vi "pulse_ring_averager.vi"() -> ()   [LabVIEW 2014]
uses:
  <vilib>/express/express analysis/Spectral/Block/exnSpectralBlock spectral measurements RMS poly.vi
  <vilib>/express/express analysis/Spectral/Block/exnSpectralBlock spectral measurements RMS WFM.vi
  <vilib>/Utility/file.llb/Write To Spreadsheet File (DBL).vi
  <vilib>/express/express analysis/Spectral/XNode/ExpressSpectralMeasurementsBlockNode.xnode
panel:
  in  "Create Spreadsheet Data?":bool
  in  "?":bool
  out "Waveform Graph":cluster{"f0":dbl, "df":dbl, "magnitude":dbl[]}(graph)={"f0"=0.0, "df"=5.0, "magnitude"=[8.352033063743602e-05, 0.0001521936782107742, 0.0001241645669166561, 0.0005913924283974822, 0.0017924539602640116, 0.002361467917160108, 0.0013264978014836787, 0.0008901875481831404, 0.00073723890923067, 0.0003785453068588639, 0.0001836739230249787, 3.197394988898929e-05, 0.00023707241273739638, 0.00018007989851456744, 4.770297439969988e-05, 0.0001260879375301181, 0.00011358993968053149, 9.416072191429606e-05, 2.3266024527903313e-05, 0.00014747301423229434, 0.00021873863503173966, 0.00016382863521811113, 0.00030989231903681013, 0.0006848998054862691, 0.0006929060488089187, 0.00011498969012903245, 0.0010445143273397997, 0.0021663414429004663, 0.0025925396298316, 0.0015150935560222308, 0.005327334532678184, 0.0233859554577817, 0.02859469559502763, 0.009897156395780392, 0.001793115328993954, 0.0005236696631654215, 0.0006446389975765783, 0.0018452938517409666, 0.0016391137319586276, 0.0005787100388248387, 0.0001698622098812452, 0.00016031383859121896, 9.318098751849772e-05, 4.9411270959326514e-05, 0.00018102626398632646, 0.0001772618334287019, 8.862654858080105e-05, 0.00010413603644766573, 4.065137938351173e-05, 6.325569194929935e-05, 3.7785144930814025e-05, 8.44451565632641e-05, 0.00011643844181054693, 0.00012102920589116524, 6.558259148383841e-05, 2.6563415271802513e-05, 9.419033683439217e-05, 0.00024452333927457243, 0.00021172954941749473, 0.00010011909206931354, 0.00040767861329374014, 0.00089963628760365, 0.0013620238335515452, 0.0033111439875997645, 0.003843956937129491, 0.0021381752402404365, 0.0006642447893147237, 0.0003523770956178529, 0.0009192108548157987, 0.00240667098631922, 0.003199856811538736, 0.0020968774819987443, 0.000781225449659328, 0.0012720686213830836, 0.0011307985420501722, 0.00041317105628617623, 5.672232242689178e-05, 0.00019255456754959516, 0.00016272162386009182, 3.994272788022854e-05, 2.911455610905325e-05, 4.3973070727008133e-05, 3.0127385533287327e-05, 5.478402759196668e-05, 7.214350960014323e-05, 0.00010803424524223192, 6.0967411444140105e-05, 5.142072772087622e-05, 4.857738287964089e-05, 0.000184071319208993, 0.00039623072384841645, 0.00037089595185725214, 0.000464718422038645, 0.0013054691711676788, 0.0015883351276961978, 0.0009090460049399212, 0.0010413359930296908, 0.0012816866380819423, 0.0010403077729971293, 0.0005914864424886577]}
  out "Dynamic Data Type":waveform(dbl)(graph)={"t0"=timestamp(0 s since 1904-01-01), "dt"=0.001, "Y"=[0.1835690300006684, -0.12360814617024107, -0.07143667530691175, -0.02653042030583372, -0.07465835397845205, 0.15772985665219794, 0.2851176340286107, -0.03432162256909273, -0.07386937144638245, -0.02297999903586587, -0.19300573901482213, 0.1247569668003238, 0.29146236688979116, 0.026002663846969525, -0.06653840876744663, -0.04457839523672956, -0.24478272315965532, 0.06269034846174756, 0.22854102520122027, 0.07031717883364498, -0.045926240368086735, -0.054769419436562515, -0.24139667270845547, -0.0006583692233529391, 0.1371176913027222, 0.09908216368629041, -0.009698793623529106, -0.05282983740577475, -0.17972453196741012, -0.0451372578516373, 0.040828959449704175, 0.1118045053650388, 0.03221590082759546, -0.03895689482236976, -0.0980648359927371, -0.06814924809680811, -0.027845391148113553, 0.10851707858601553, 0.06393957068076692, -0.022191016532421108, -0.026398923220259607, -0.0778471583886443, -0.03083694982363553, 0.09776719296298968, 0.08442024005246113, -0.0028938196171412545, 0.01189960202745971, -0.08212081379058926, -0.0309355726361973, 0.07534694194051353, 0.09007461420853317, 0.01906619290029264, -0.007824960198172675, -0.08087159144056387, -0.04740558259182132, 0.04622033962280515, 0.08185604711414643, 0.03842913777594848, -0.023341616025494043, -0.07288314329513075, -0.06755751120093278, 0.011373613704546709, 0.06430118763381847, 0.05434028412241818, -0.007792085929768459, -0.05638025875261071, -0.06900397917255532, -0.023867604355561515, 0.040270096868167723, 0.057693459576050155, 0.01883607301247459, -0.03402575413089732, -0.053980436925205544, -0.043296298651859515, 0.020085295269852928, 0.05647711162085163, 0.036785424301965415, -0.006838732080940968, -0.04138959090587689, -0.056676127198896996, -6.663235528466547e-05, 0.04881740690551869, 0.042867164154510556, 0.015187029038378999, -0.02695778583040371, -0.054900916522599555, -0.014268317253597385, 0.03408973419593303, 0.039152371704780406, 0.026232783736334912, -0.017325624439389554, -0.03954863171291109, -0.020021314656622283, 0.020282540889840796, 0.03668680148402867, 0.027679251601125072, -0.011506878517493845, -0.02945623043904346, -0.02639892323035415, 0.00762594690151389, 0.03507596228025529, 0.025706795413523692, -0.002565076913941361, -0.02646467176420441, -0.03238204057229209, -0.006707235002267768, 0.026561526434138838, 0.02481919012914729, 0.009697025920002537, -0.01916658360774865, -0.03057395565343716, -0.017128378819227883, 0.014332298014551614, 0.026232783732030158, 0.01620613140665912, -0.008416697070999096, -0.02722077999814542, -0.02271700486985124, 0.004075525709689282, 0.025673921148851364, 0.019888049649393853, 0.00026211034925005457, -0.023045747576780858, -0.02274987913918223, -0.0020062143120944662, 0.022616614052667332, 0.025378052720173495, 0.008579300738602344, -0.016569516210291884, -0.02495245529686407, -0.010224781957309206, 0.012721458782050842, 0.025509549800730967, 0.01531852611708286, -0.006575737916810642, -0.02117191413339948, -0.014925802669450403, 0.0019386981387649702, 0.019427809871566372, 0.01577876590018839, 0.0014455840833056948, -0.014399814337060024, -0.01673388756407459, -0.0032883108599840102, 0.013050201482682548, 0.01558152028048325, 0.005489119336503034, -0.010619273205090617, -0.01604352787783086, -0.006214120939702474, 0.008447803659105033, 0.015351400388196152, 0.008184809496223239, -0.007463343221417863, -0.015517539544145188, -0.009830290708467831, 0.0037139087382661224, 0.014924034879149164, 0.011373613706054674, -0.001315854634032015, -0.012854723610625044, -0.012657477986467363, -0.0006583692231487726, 0.011011996735723395, 0.012557087432060937, 0.0035824116580306506, -0.008778314046058, -0.011967118301432666, -0.0026965739916566243, 0.006836964418459937, 0.011340739436402255, 0.005916484848471818, -0.004603281682111682, -0.010783644556400252, -0.005096395740947415, 0.0042398970650034794, 0.010453134142121378, 0.007494449823131834, -0.0024664540985765383, -0.00871256550526097, -0.008975559670553301, 0.0006237273240890565, 0.009006666253500255, 0.009335408953810034, 0.0017085782461639186, -0.006575737915334561, -0.009863164978560159, -0.004208790436638608, 0.004634388308552668, 0.00946690603627583, 0.0051932509032384215, -0.002663699721996195, -0.008022205821129115, -0.004636155952486639, 0.0007223501350646876, 0.00706708431025217, 0.00473301111953617, -0.0008227405745680856, -0.005523761256395014, -0.004701904493299368]}
  in  "rate":dbl=1000.0
  in  "seconds to wait":dbl=0.2
  in  "Averages":i32=10
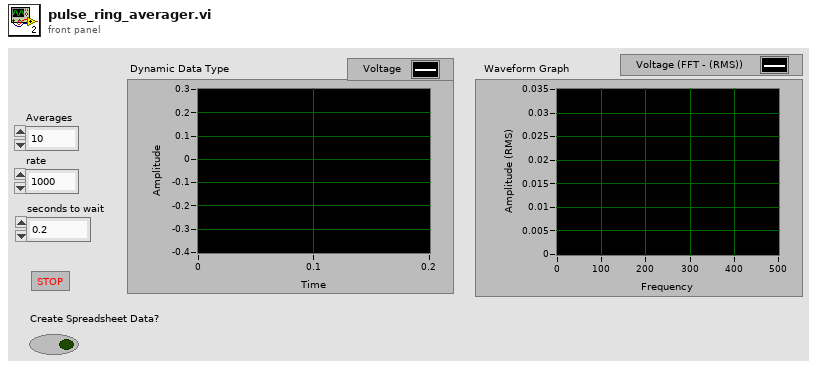
[diagram p1: front panel]
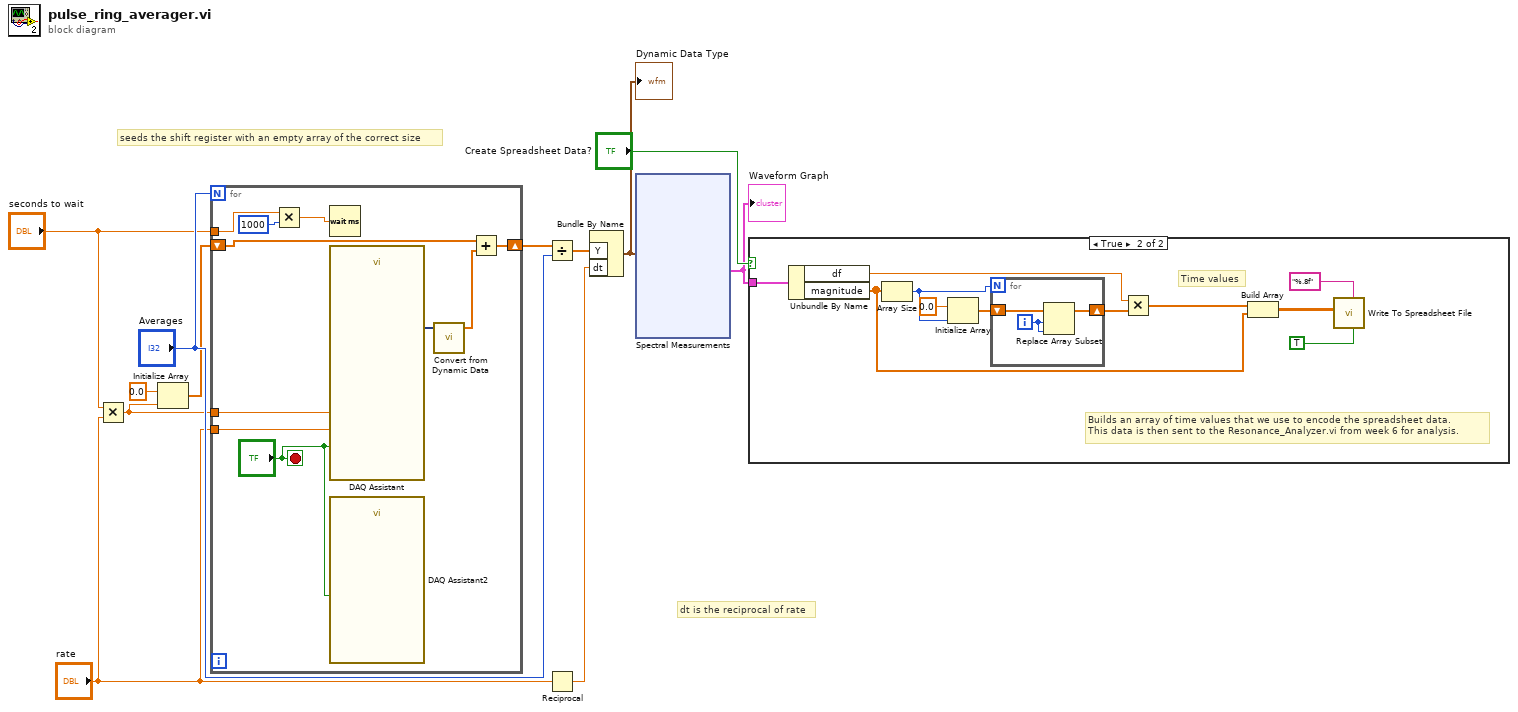
[diagram p0: block diagram]
diagram:
  # "seeds the shift register with an empty array of the correct size"
  # "dt is the reciprocal of rate"
  n1 = Multiply(x="seconds to wait", y="rate") -> (x*y=w9:dbl)
  n2 = Initialize Array(0.0 ("element"), w9) -> (w7:dbl[])
  n3 = for {
    N: "Averages" -> [_]
    shift-right: [w17] -> w11
    shift-left: w7 -> [w20]
    tunnel: w9 -> [w16]
    tunnel: "seconds to wait" -> [w15]
    tunnel: "rate" -> [w14]
    stop <- "?" stop-if-true
    n4 = Multiply(x=w15, y=1000) -> (x*y=w21:dbl)
    n5 = Wait (ms)(milliseconds to wait=w21) -> ()  [unwired: 1 out]
    n6 = call "DAQ Assistant"("rate"=w14, "number of samples"=w16, "stop (T)"="?") -> ("data"=w19:dynamicdata)  [unwired: 14 in, 2 out]
    n7 = call "DAQ Assistant2"("stop (T)"="?") -> ()  [unwired: 17 in, 2 out]
    n8 = call "Convert from Dynamic Data"("Dynamic Data Type"=w19) -> ("Array"=w18:dbl[])  [unwired: 3 in]
    n9 = Add(x=w20, y=w18) -> (x+y=w17:dbl[])
  }
  n10 = Divide(x=w11, y="Averages") -> (x/y=w6:dbl[])
  n11 = Reciprocal(x="rate") -> (1/x=w4:dbl)
  n12 = Bundle By Name("Y"=w6, "dt"=w4) -> (w3:waveform(dbl))  [unwired: 1 in]
  "Dynamic Data Type" <- w3
  n13 = xnode "Spectral Measurements"("Signals"=w3) -> ("FFT - (RMS)"=w1:cluster{"f0":dbl, "df":dbl, "magnitude":dbl[]})  [unwired: 1 in, 2 out]
  "Waveform Graph" <- w1
  n14 = case shown="True" "Create Spreadsheet Data?" {
    tunnel: w1 -> [_ w28]
    frame False {
    }
    frame True {
      # "Time values"
      # "Builds an array of time values that we use to encode the spreadsheet data. \nThis data is then sent to the Resonance_Analyzer.vi from week 6 for analysis."
      n15 = Unbundle By Name(w28) -> ("df"=w31:dbl, "magnitude"=w26:dbl[])
      n16 = Array Size(array=w26) -> (size(s)=w29:i32)
      n17 = Initialize Array(0.0 ("element"), w29) -> (w32:dbl[])
      n18 = for {
        N: w29 -> [_]
        shift-right: [w34] -> w33
        shift-left: w32 -> [w35]
        i -> [w36]
        n19 = Replace Array Subset(array=w35, new element=w36, index=w36) -> (w34:dbl[])
      }
      n20 = Multiply(x=w31, y=w33) -> (x*y=w27:dbl[])
      n21 = Build Array(w27, w26) -> (w25:dbl[][])
      n22 = call-poly <vilib>:"Write To Spreadsheet File.vi"("transpose? (no:F)"=TRUE, "format (%.3f)"="%.8f", "2D data"=w25) -> ()  [unwired: 5 in, 1 out]
    }
  }
